vi "CameraCheckROI.vi"(8 "error in (no error)":errorcluster, 10 "ROI_in":T1, 11 "Photonfocus in":refnum<class "Photonfocus.lvclass">) -> (0 "error out":errorcluster, 2 "ROI_out":T1, 3 "Photonfocus out":refnum<class "Photonfocus.lvclass">)   [LabVIEW 2010, in "Photonfocus.lvclass"]
uses:
  Photonfocus.lvclass
  subvis/ROI_rect.ctl
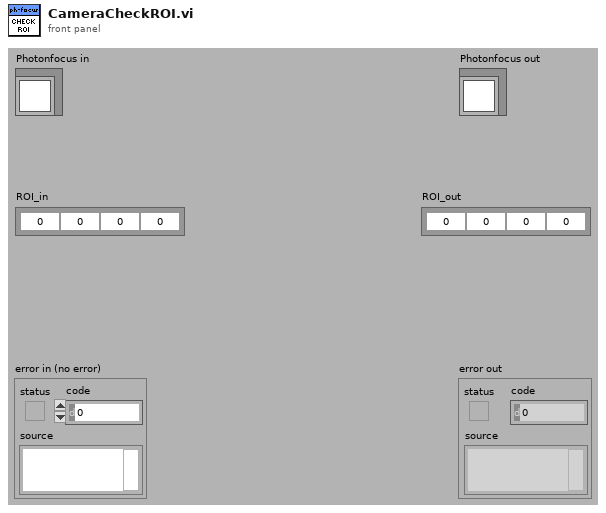
[diagram p1: front panel]
types:
  T1 = typedef "ROI_rect.ctl" = cluster{"left":i32, "top":i32, "right":i32, "bottom":i32}
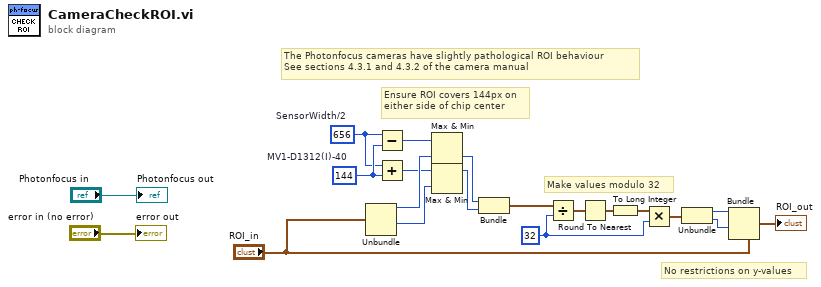
[diagram p0: block diagram]
diagram:
  w9 = 32
  w15 = 656  # SensorWidth/2
  w16 = 144  # MV1-D1312(I)-40
  # "No restrictions on y-values"
  # "Make values modulo 32"
  # "Ensure ROI covers 144px on\neither side of chip center"
  # "The Photonfocus cameras have slightly pathological ROI behaviour\nSee sections 4.3.1 and 4.3.2 of the camera manual"
  n1 = Unbundle("ROI_in") -> ("left"=w18:i32, "right"=w13:i32)  [unwired: 2 out]
  n2 = Subtract(x=w15, y=w16) -> (x-y=w17:i32)
  n3 = Add(x=w15, y=w16) -> (x+y=w14:i32)
  n4 = Max & Min(x=w17, y=w18) -> (min(x,y)=w12:i32)  [unwired: 1 out]
  n5 = Max & Min(x=w14, y=w13) -> (max(x,y)=w6:i32)  [unwired: 1 out]
  n6 = Bundle(w12, w6) -> (w11:cluster{i32, i32})  [unwired: 1 in]
  n7 = Divide(x=w11, y=w9) -> (x/y=w10:cluster{dbl, dbl})
  n8 = Round To Nearest(number=w10) -> (nearest integer value=w8:cluster{dbl, dbl})
  n9 = To Long Integer(number=w8) -> (32bit integer=w7:cluster{i32, i32})
  n10 = Multiply(x=w7, y=w9) -> (x*y=w5:cluster{i32, i32})
  n11 = Unbundle(w5) -> (w3:i32, w2:i32)
  n12 = Bundle(cluster="ROI_in", "left"=w3, "right"=w2) -> (→"ROI_out":T1)  [unwired: 2 in]
  "error out" <- "error in (no error)"
  "Photonfocus out" <- "Photonfocus in"
